vi "acquireORCAImageHDR.vi"(4 "error in (no error)":errorcluster {"code" format="%.0x"}, 7 "Handle in":u32) -> (0 "error out":errorcluster {"code" format="%.0x"}, 2 "Image":u16[][](graph), 3 "Handle out":u32)   [LabVIEW 2016]
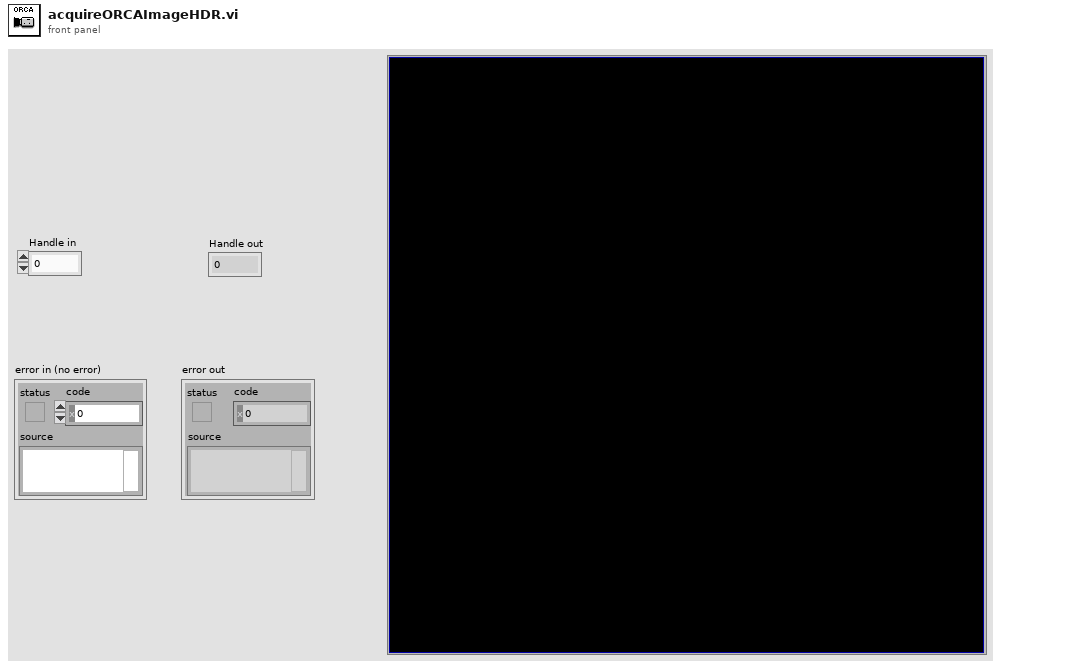
[diagram p1: front panel]
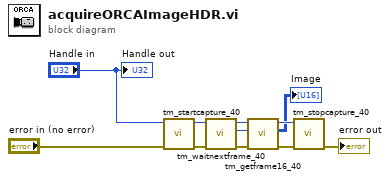
[diagram p0: block diagram]
diagram:
  n1 = call <userlib>:"tm_startcapture_40.vi"("error in (no error)"="error in (no error)", "Handle in"="Handle in") -> ("error out"=w7:errorcluster, "Handle out"=w6:u32)  [unwired: 8 in]
  n2 = call <userlib>:"tm_waitnextframe_40.vi"("error in (no error)"=w7, "Handle in"=w6) -> ("error out"=w3:errorcluster, "Frame Index"=w4:i32, "Handle out"=w5:u32)  [unwired: 6 in, 1 out]
  n3 = call <userlib>:"tm_getframe16_40.vi"("error in (no error)"=w3, "Frame Index"=w4, "Handle in"=w5) -> ("error out"=w10:errorcluster, "Data"=→"Image":u16[][], "Handle out"=w11:u32)  [unwired: 5 in, 1 out]
  n4 = call <userlib>:"tm_stopcapture_40.vi"("error in (no error)"=w10, "Handle in"=w11) -> ("error out"=→"error out":errorcluster)  [unwired: 8 in, 1 out]
  "Handle out" <- "Handle in"
